vi "set_physical_channel.vi"(8 "error in (no error)":errorcluster, 10 "physical channel":tag, 11 "DAQmxWriteSignals.lvclass in":refnum<class "SignalWriterMM140725DAQmx.lvclass">) -> (0 "error out":errorcluster, 3 "DAQmxWriteSignals.lvclass out":refnum<class "SignalWriterMM140725DAQmx.lvclass">)   [LabVIEW 2010, in "SignalWriterMM140725DAQmx.lvclass"]
uses:
  SignalWriterMM140725DAQmx.lvclass
  SignalWriterMM140725DAQmx.lvclass/SignalWriterMM140725DAQmx.ctl
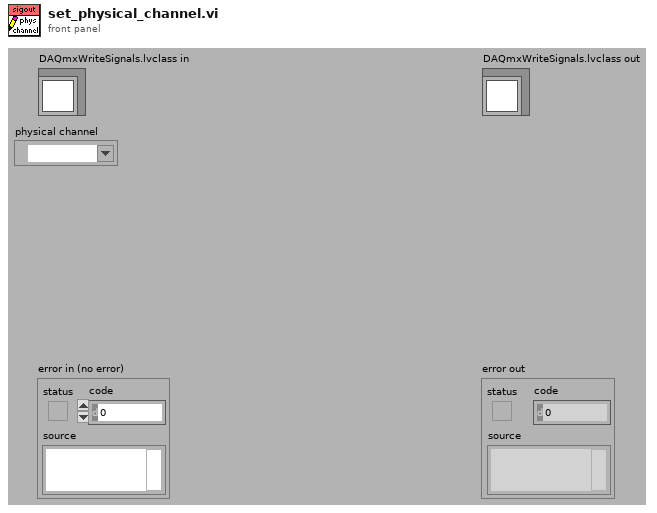
[diagram p1: front panel]
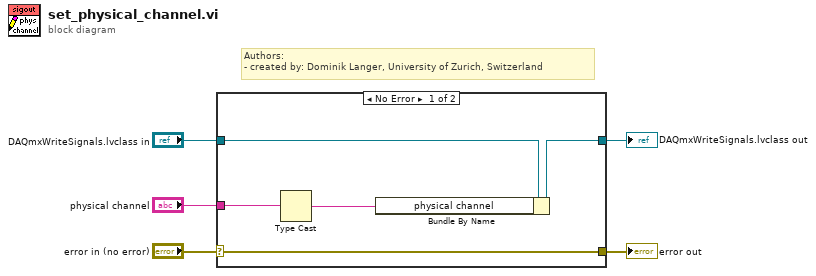
[diagram p0: block diagram]
diagram:
  # "Authors: \n- created by: Dominik Langer, University of Zurich, Switzerland"
  n1 = case shown="No Error" "error in (no error)" {
    selector: "error in (no error)" -> [w10 w11]
    tunnel: [w10 w11] -> w4
    tunnel: [w8 w12] -> w2
    tunnel: "DAQmxWriteSignals.lvclass in" -> [w9 w12]
    tunnel: "physical channel" -> [w7 _]
    frame No Error {
      n2 = Type Cast(x=w7) -> (*(type *) &x=w6:string)  [unwired: 1 out]
      n3 = Bundle By Name(cluster=w9, "physical channel"=w6) -> (w8:refnum<class "SignalWriterMM140725DAQmx.lvclass">)
    }
    frame Error {
    }
  }
  "error out" <- w4
  "DAQmxWriteSignals.lvclass out" <- w2
